vi "Edge Detection (FPGA).vi"(2 "Mask End Angle":fxp<+/-,32,16>, 3 "Mask Start Angle":fxp<+/-,32,16>, 4 "Mean Pixel Values By Sector":fxp<+/-,32,16>[](array[numeric])) -> (0 "Edge Angle":fxp<+/-,32,16>, 1 "Edge Sector":u8)   [LabVIEW 2013, in "FPGA Image Processing.lvlib"]
uses:
  FPGA Image Processing.lvlib
panel:
  out "numSectors":i32
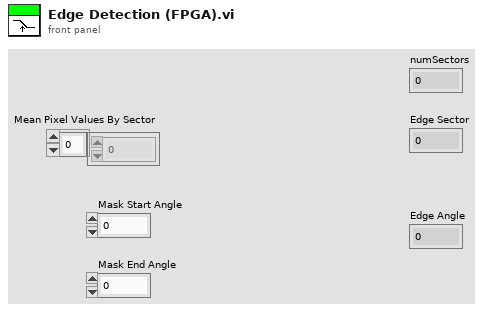
[diagram p1: front panel]
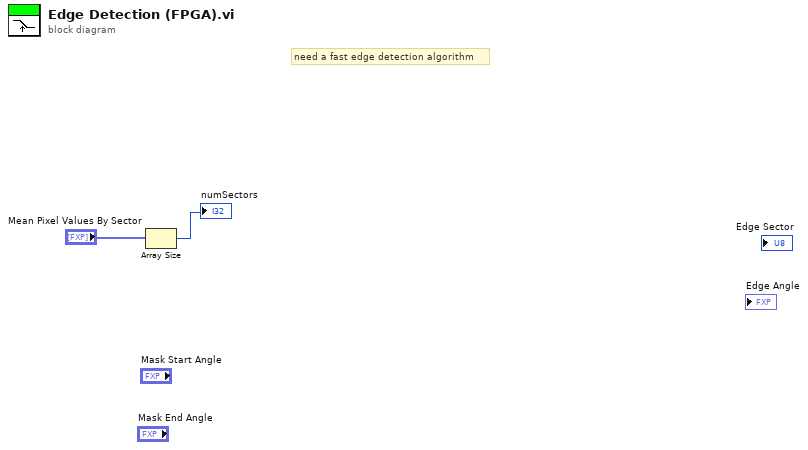
[diagram p0: block diagram]
diagram:
  # "need a fast edge detection algorithm"
  n1 = Array Size(array="Mean Pixel Values By Sector") -> (size(s)=→"numSectors":i32)
